vi "电池信息全局变量.vi"() -> ()   [LabVIEW 2013]
panel:
  out "Rly":u8
  out "BMS_Volt":dbl
  out "充电":dbl
  out "预充":dbl
  out "总负":dbl
  out "总正":dbl
  out "允许保存数据":bool
  out "刷新计数":dbl
  out "DI_D":u8
  out "DO_D":u8
  out "CC2":dbl
  out "CC":dbl
  out "CP":u8
  out "电池信息解析2":string[](array[string])
  out "硬件故障":string[](array[string])
  out "其他故障":string[](array[string])
  out "电池系统故障":string[](array[string])
  out "电池故障":string[](array[string])
  out "充电机累计输出能量":dbl
  out "充电机输出电流":dbl
  out "充电机输出电压":dbl
  out "最高允许充电温度":dbl
  out "充电电流步长":dbl
  out "最小允许充电电流":dbl
  out "最大允许充电电流":dbl
  out "最高允许充电单体电压":dbl
  out "最高允许充电总电压":dbl
  out "剩余充电时间":dbl
  out "累计充电时间":dbl
  out "列1":dbl[](array[numeric])
  out "F":dbl[](array[numeric])
  out "10":string[](array[string])
  out "07":dbl
  out "从板个数":dbl
  out "电池信息解析":dbl[](array[numeric])
  out "功率":dbl
  out "负绝缘":dbl
  out "正绝缘":dbl
  out "DI":string[](array[string])
  out "DO":string[](array[string])
  out "AI2":dbl
  out "AI1":dbl
  out "辅助继电器B":dbl
  out "辅助继电器A":dbl
  out "放电总安时":dbl
  out "充电总安时":dbl
  out "实际容量":dbl
  out "最大放电电流":dbl
  out "最大充电电流":dbl
  out "平均电流":dbl
  out "外总压":dbl
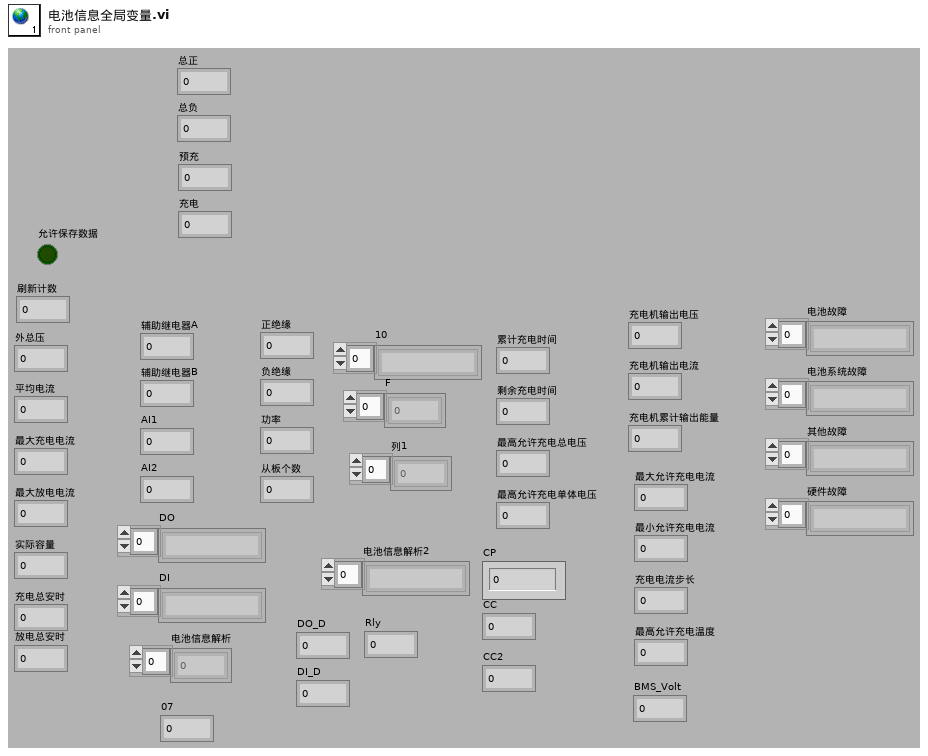
[diagram p1: front panel]
diagram:
